vi "f_ON_Region.vi"(0 "VISA Resource Name":refnum<visa-resource-name>, 1 "Project #":string, 2 "Request #":string, 3 "TEST #":string, 4 "ICE":dbl, 5 "VGE":dbl, 6 "VCE":dbl, 7 "error in (no error)":errorcluster) -> (8 "Tdon (ns)":dbl, 9 "Di (A)":dbl, 10 "Tr (ns)":dbl, 11 "Dt (ns)":dbl, 12 "Di/Dt (A/us)":dbl, 14 "Dv/Dt (V/us)":dbl, 16 "Eon (uj)":dbl, 17 "Dv (V)":dbl, 19 "Dt (ns) 2":dbl, 20 "DONE Tdon":bool, 21 "DONE Tr":bool, 22 "DONE Di/Dt ON":bool, 23 "DONE Dv/Dt ON":bool, 24 "DONE Eon":bool, 25 "Oscilloscope Capture":waveform(dbl)[](graph), 27 "error out":errorcluster)   [LabVIEW 2020]
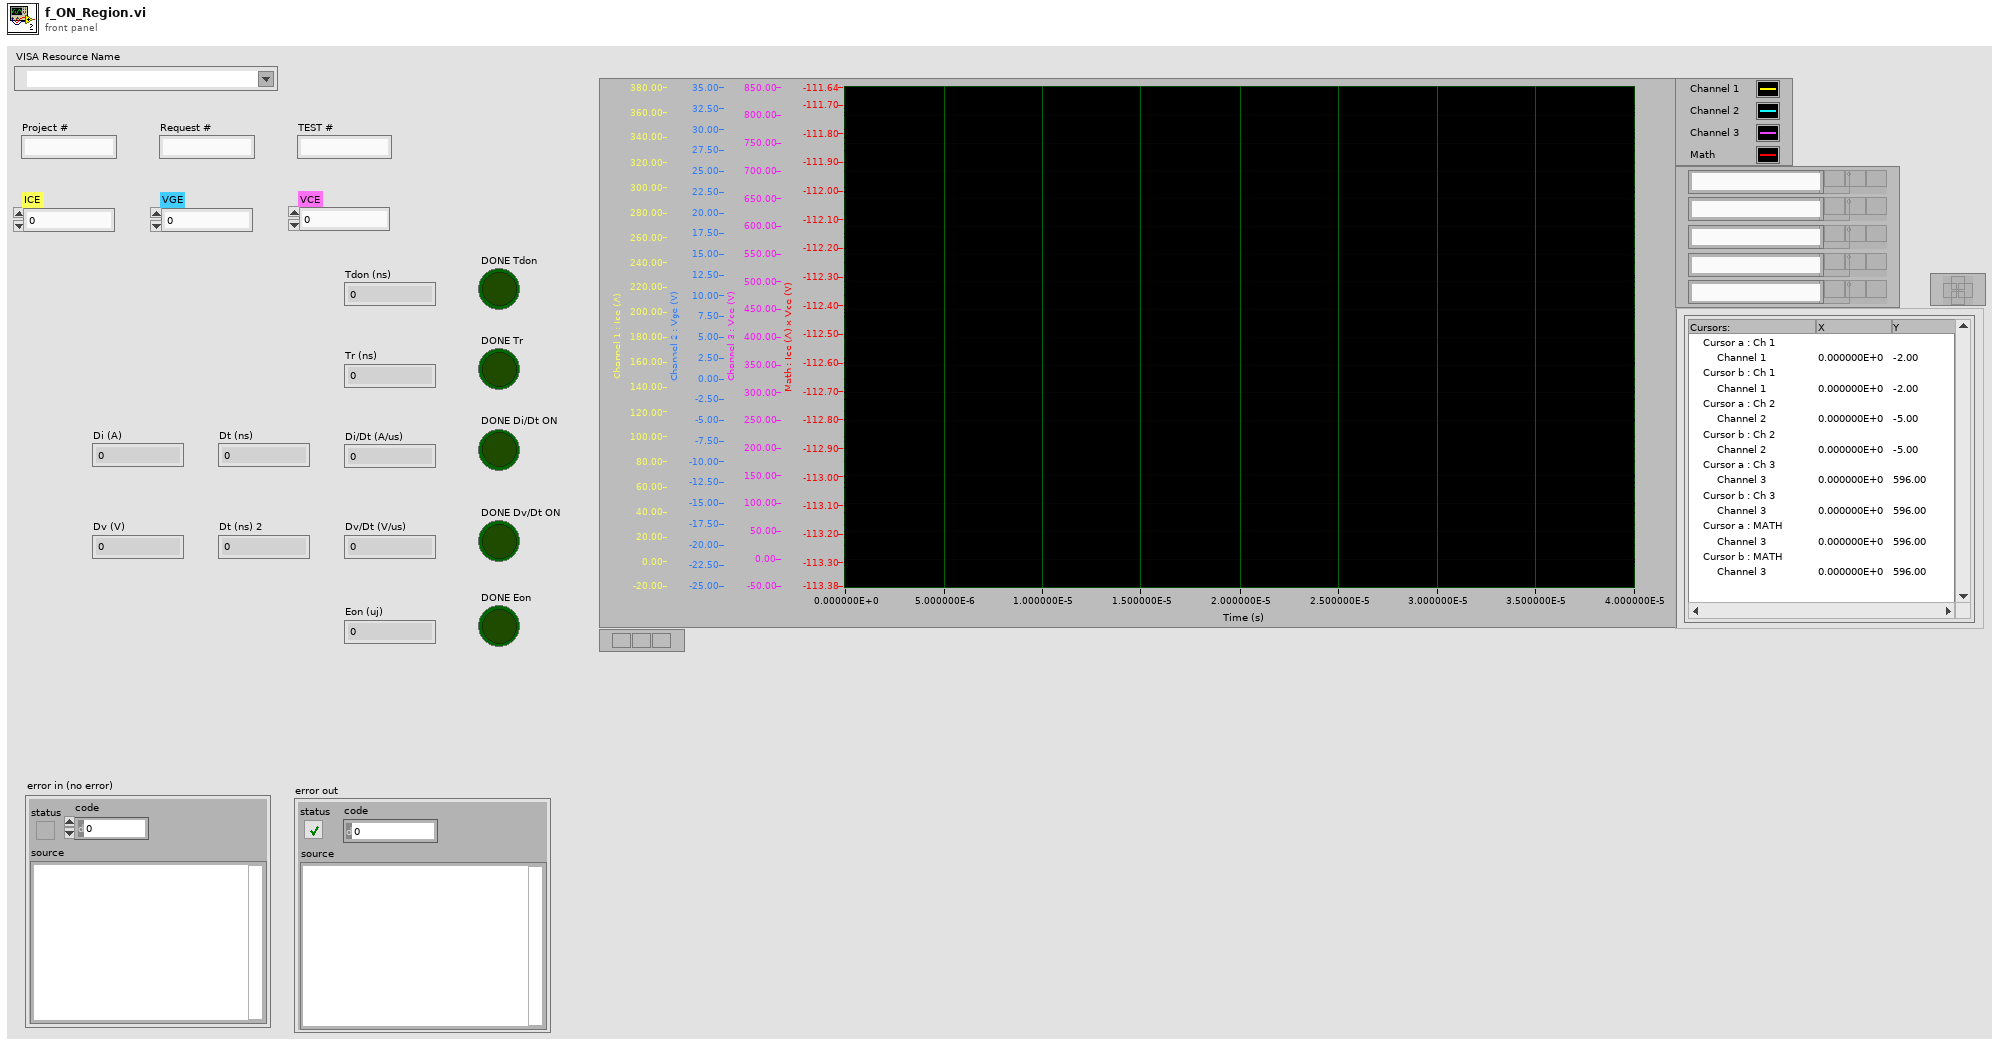
[diagram p1: front panel]
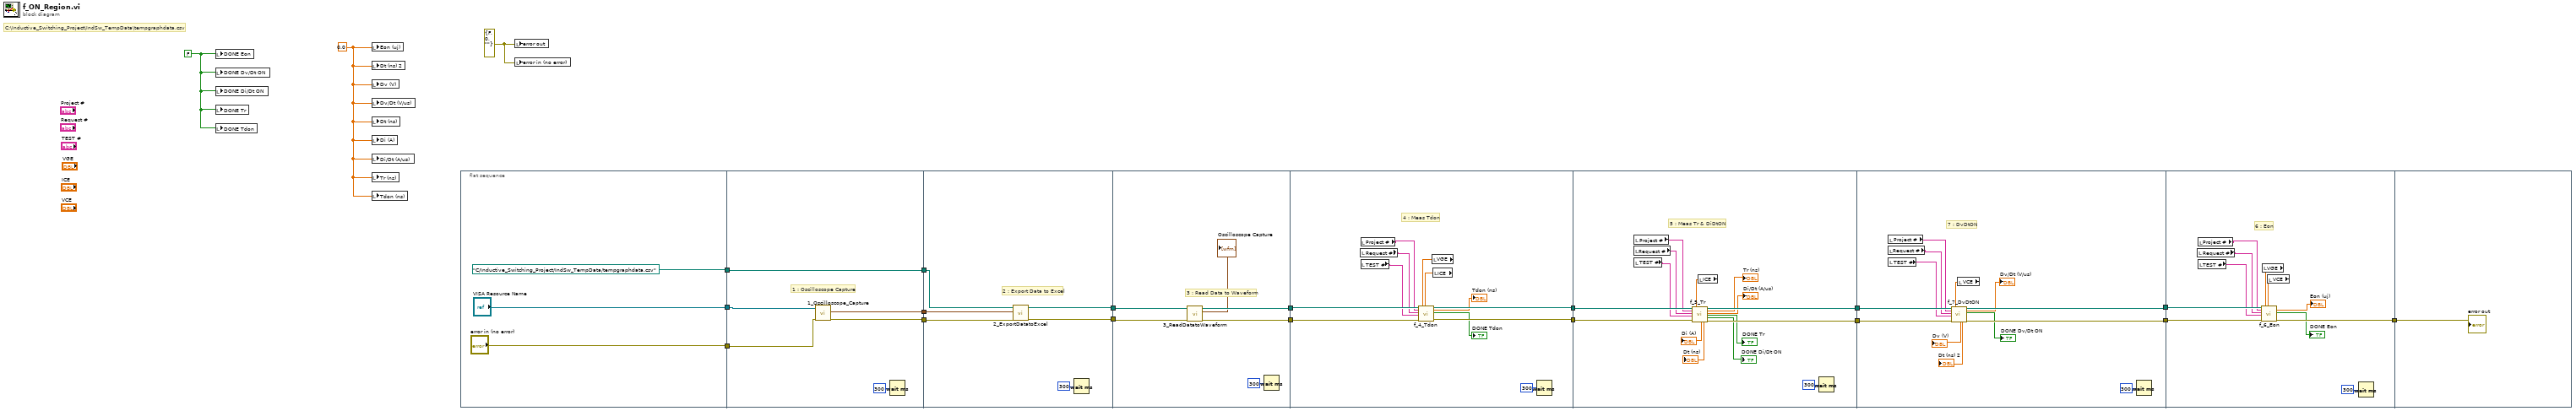
[diagram p0: block diagram]
diagram:
  w3 = errorcluster {"status"=FALSE, "code"=0, "source"=""} ("error out")
  w4 = 0.0 ("Eon (uj)")
  w5 = FALSE ("DONE Eon")
  # "C:\\Inductive_Switching_Project\\IndSw_TempData\\tempgraphdata.csv"
  n1 = local write "DONE Eon"(w5) -> ()
  n2 = local write "DONE Dv/Dt ON"(w5) -> ()
  n3 = local write "DONE Di/Dt ON"(w5) -> ()
  n4 = local write "DONE Tr"(w5) -> ()
  n5 = local write "DONE Tdon"(w5) -> ()
  n6 = local write "Eon (uj)"(w4) -> ()
  n7 = local write "Dt (ns) 2"(w4) -> ()
  n8 = local write "Dv (V)"(w4) -> ()
  n9 = local write "Dv/Dt (V/us)"(w4) -> ()
  n10 = local write "Dt (ns)"(w4) -> ()
  n11 = local write "Di (A)"(w4) -> ()
  n12 = local write "Di/Dt (A/us)"(w4) -> ()
  n13 = local write "Tr (ns)"(w4) -> ()
  n14 = local write "Tdon (ns)"(w4) -> ()
  n15 = flat-sequence {
    tunnel: [path "C:/Inductive_Switching_Project/IndSw_TempData/tempgraphdata.csv" ("file path (IN)")] -> w20
    tunnel: ["error in (no error)"] -> w19
    tunnel: ["VISA Resource Name"] -> w18
    tunnel: [w26] -> w17
    tunnel: [w25] -> w16
    tunnel: [w29] -> w15
    tunnel: w20 -> [w29]
    tunnel: w19 -> [w28]
    tunnel: w18 -> [w27]
    tunnel: [w32] -> w14
    tunnel: [w31] -> w13
    tunnel: w17 -> [w35]
    tunnel: w16 -> [w34]
    tunnel: w15 -> [w33]
    tunnel: [w39] -> w2
    tunnel: [w38] -> w1
    tunnel: w14 -> [w41]
    tunnel: w13 -> [w40]
    tunnel: [w49] -> w12
    tunnel: [w51] -> w11
    tunnel: w2 -> [w52]
    tunnel: w1 -> [w50]
    tunnel: [w65] -> w10
    tunnel: [w64] -> w9
    tunnel: w12 -> [w67]
    tunnel: w11 -> [w66]
    tunnel: [w78] -> w8
    tunnel: [w77] -> w7
    tunnel: w10 -> [w79]
    tunnel: w9 -> [w80]
    tunnel: [w89] -> w6
    tunnel: w8 -> [w91]
    tunnel: w7 -> [w90]
    tunnel: w6 -> [w93]
    frame #0 {
    }
    frame #1 {
      # "1 : Oscilloscope Capture"
      n16 = call "1_Oscilloscope_Capture.vi"("error in (no error)"=w28, "VISA Resource Name"=w27) -> ("error out"=w26:errorcluster, "Waveform Graph"=w25:waveform(dbl)[])  [unwired: 7 in, 1 out]
      n17 = Wait (ms)(milliseconds to wait=u32 300) -> ()  [unwired: 1 out]
    }
    frame #2 {
      # "2 : Export Data to Excel"
      n18 = call "2_ExportDatatoExcel.vi"("error in (no error)"=w35, "Waveform Graph"=w34, "file path (IN)"=w33) -> ("error out"=w32:errorcluster, "file path (OUT)"=w31:path)  [unwired: 7 in]
      n19 = Wait (ms)(milliseconds to wait=u32 300) -> ()  [unwired: 1 out]
    }
    frame #3 {
      # "3 : Read Data to Waveform"
      n20 = call "3_ReadDatatoWaveform.vi"("error in (no error)"=w41, "file path (IN)"=w40) -> ("error out"=w39:errorcluster, "Waveform Graph"=→"Oscilloscope Capture":waveform(dbl)[], "file path (OUT)"=w38:path)  [unwired: 3 in, 4 out]
      n21 = Wait (ms)(milliseconds to wait=u32 300) -> ()  [unwired: 1 out]
    }
    frame #4 {
      # "4 : Meas Tdon"
      n22 = local read "Request #"() -> (w45:string)
      n23 = local read "Project #"() -> (w46:string)
      n24 = local read "TEST #"() -> (w44:string)
      n25 = local read "VGE"() -> (w48:dbl)
      n26 = local read "ICE"() -> (w47:dbl)
      n27 = call "f_4_Tdon.vi"("file path (IN)"=w50, "Project #"=w46, "Request #"=w45, "TEST #"=w44, "error in (no error)"=w52, "VGE"=w48, "ICE"=w47) -> ("file path (OUT)"=w49:path, "Tdon (ns) (after filter)"=→"Tdon (ns)":dbl, "DONE Tdon"=→"DONE Tdon":bool, "error out"=w51:errorcluster)  [unwired: 9 in]
      n28 = Wait (ms)(milliseconds to wait=u32 300) -> ()  [unwired: 1 out]
    }
    frame #5 {
      # "5 : Meas Tr & DiDtON"
      n29 = local read "Request #"() -> (w62:string)
      n30 = local read "Project #"() -> (w63:string)
      n31 = local read "TEST #"() -> (w61:string)
      n32 = local read "ICE"() -> (w60:dbl)
      n33 = call "f_5_Tr.vi"("file path (IN)"=w67, "Project #"=w63, "Request #"=w62, "TEST #"=w61, "error in (no error)"=w66, "ICE"=w60) -> ("Di (A)"=→"Di (A)":dbl, "Dt (ns)"=→"Dt (ns)":dbl, "file path (OUT)"=w65:path, "Tr (ns)"=→"Tr (ns)":dbl, "Di/Dt (A/us)"=→"Di/Dt (A/us)":dbl, "DONE Tr"=→"DONE Tr":bool, "DONE Di/Dt ON"=→"DONE Di/Dt ON":bool, "error out"=w64:errorcluster)  [unwired: 6 in]
      n34 = Wait (ms)(milliseconds to wait=u32 300) -> ()  [unwired: 1 out]
    }
    frame #6 {
      # "7 : DvDtON"
      n35 = local read "Request #"() -> (w75:string)
      n36 = local read "Project #"() -> (w76:string)
      n37 = local read "TEST #"() -> (w74:string)
      n38 = local read "VCE"() -> (w73:dbl)
      n39 = call "f_7_DvDtON.vi"("file path (IN)"=w79, "Project #"=w76, "Request #"=w75, "TEST #"=w74, "error in (no error)"=w80, "VCE"=w73) -> ("Dv (V)"=→"Dv (V)":dbl, "Dt (ns)"=→"Dt (ns) 2":dbl, "file path (OUT)"=w78:path, "Dv/Dt (V/us)"=→"Dv/Dt (V/us)":dbl, "DONE Dv/Dt ON"=→"DONE Dv/Dt ON":bool, "error out"=w77:errorcluster)  [unwired: 8 in]
      n40 = Wait (ms)(milliseconds to wait=u32 300) -> ()  [unwired: 1 out]
    }
    frame #7 {
      # "6 : Eon"
      n41 = local read "Request #"() -> (w87:string)
      n42 = local read "Project #"() -> (w88:string)
      n43 = local read "TEST #"() -> (w86:string)
      n44 = local read "VGE"() -> (w85:dbl)
      n45 = local read "VCE"() -> (w84:dbl)
      n46 = call "f_6_Eon.vi"("file path (IN)"=w91, "Project #"=w88, "Request #"=w87, "TEST #"=w86, "error in (no error)"=w90, "VGE"=w85, "VCE"=w84) -> ("Eon (uj)"=→"Eon (uj)":dbl, "DONE Eon"=→"DONE Eon":bool, "error out"=w89:errorcluster)  [unwired: 9 in, 1 out]
      n47 = Wait (ms)(milliseconds to wait=u32 300) -> ()  [unwired: 1 out]
    }
    frame #8 {
      "error out" <- w93
    }
  }
  n48 = local write "error out"(w3) -> ()
  n49 = local write "error in (no error)"(w3) -> ()
